vi "item_to_string.vi"(8 "error in (no error)":errorcluster, 10 "Item in":refnum<class "Item.lvclass">) -> (0 "error out":errorcluster, 2 "string_value":string)   [LabVIEW 2020, in "toml.lvclass"]
uses:
  toml.lvclass
  Item/Item.lvclass
  Value/Value.lvclass
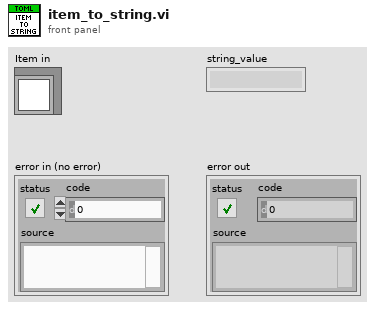
[diagram p1: front panel]
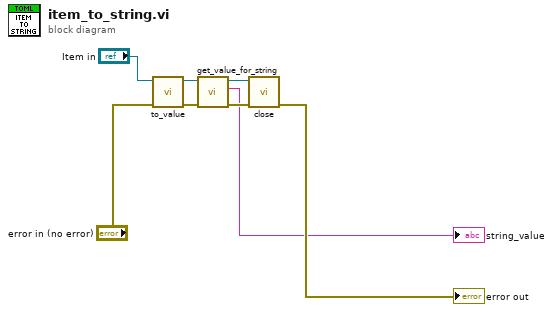
[diagram p0: block diagram]
diagram:
  n1 = call "to_value.vi"("error in (no error)"="error in (no error)", "Item in"="Item in") -> ("error out"=w2:errorcluster, "Value out"=w1:refnum<class "Value.lvclass">)  [unwired: 8 in]
  n2 = call "get_value_for_string.vi"("error in (no error)"=w2, "Value in"=w1) -> ("error out"=w5:errorcluster, "string_value"=→"string_value":string, "Value out"=w4:refnum<class "Value.lvclass">)  [unwired: 7 in]
  n3 = call "close.vi"("error in (no error)"=w5, "Value in"=w4) -> ("error out"=→"error out":errorcluster)  [unwired: 9 in]
